vi "GOTO SL DW Test.vi"(2 "Error In (no error)":errorcluster, 3 "Set Wavelength":dbl min=0.0 max=2000.0 format="%.3f", 4 "Resource Name":refnum<visa-resource-name>="ASRL1::INSTR") -> (0 "Error Out":errorcluster, 1 "Resource Name 2":refnum<visa-resource-name>="ASRL1::INSTR")   [LabVIEW 2017]
panel:
  out "Bytes in Port":u32
  out "Read String":string
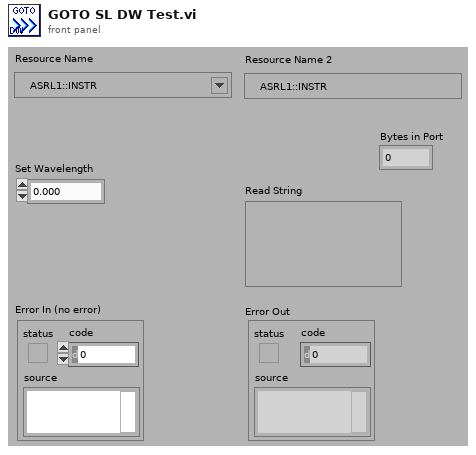
[diagram p1: front panel]
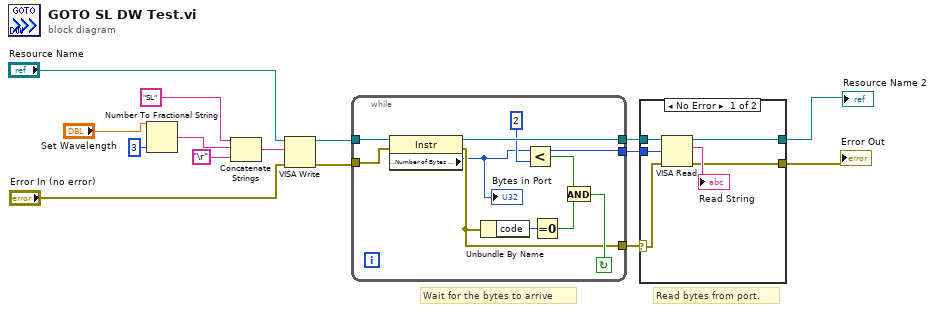
[diagram p0: block diagram]
diagram:
  # "Read bytes from port."
  # "Wait for the bytes to arrive"
  n1 = Number To Fractional String(number="Set Wavelength", precision (6)=3) -> (F-format string=w10:string)  [unwired: 2 in]
  n2 = Concatenate Strings("SL" ("SL"), w10, "\r") -> (w12:string)
  n3 = VISA Write(VISA resource name="Resource Name", write buffer=w12, error in (no error)="Error In (no error)") -> (VISA resource name out=w2:refnum<visa-resource-name>, error out=w1:errorcluster)  [unwired: 1 out]
  n4 = while {
    tunnel: [w18] -> w8
    tunnel: [w16] -> w7
    tunnel: w2 -> [w24]
    tunnel: w1 -> [w19]
    tunnel: [w25] -> w9
    stop <- w21 continue-if-true
    n5 = property class="Instr"(reference=w24, error in=w19) -> (reference out=w25:refnum<visa-resource-name>, error out=w18:errorcluster, "Serial Settings:Number of Bytes at Serial Port"=w16:u32)
    "Bytes in Port" <- w16
    n6 = Unbundle By Name(w18) -> ("code"=w20:i32)
    n7 = Less?(x=w16, y=u32 2 ("Bytes to Read")) -> (x < y?=w23:bool)
    n8 = Equal To 0?(x=w20) -> (x = 0?=w22:bool)
    n9 = And(x=w23, y=w22) -> (x .and. y?=w21:bool)
  }
  n10 = case "Read bytes from port." shown="No Error" w8 {
    selector: w8 -> [w27 w32]
    tunnel: [w30 w32] -> w5
    tunnel: w9 -> [w29 w33]
    tunnel: w7 -> [w28 _]
    tunnel: [w26 w33] -> w6
    frame No Error {
      n11 = VISA Read(VISA resource name=w29, byte count=w28, error in (no error)=w27) -> (VISA resource name out=w26:refnum<visa-resource-name>, read buffer=→"Read String":string, error out=w30:errorcluster)  [unwired: 1 out]
    }
    frame Error {
      # "Error occurred \nreading Bytes at \nSerial Port"
    }
  }
  "Error Out" <- w5
  "Resource Name 2" <- w6
